vi "Stopped.vi"(6 "Teller":refnum<class "Teller.lvclass">, 8 "Error in":errorcluster, 9 "Error":errorcluster, 10 "Actor":refnum<class "Actor.lvclass">, 11 "Base Actor in":refnum<class "Base Actor.lvclass">) -> (0 "Error out":errorcluster, 3 "Base Actor out":refnum<class "Base Actor.lvclass">)   [LabVIEW 2025, in "jettl.lvlib" / "Base Actor.lvlib" / "Base Actor.lvclass"]
uses:
  Base Actor.lvclass
  C:/git/jettl/src/jettl/jettl/Actor/Actor.lvclass
  Actor/Actor.lvclass
  Teller/Teller.lvclass
  Base Actor.lvclass/Base Actor.ctl
  Stop jettl Msg/Call.vi
  Attributes/Attributes.lvclass
  C:/git/jettl/src/jettl/jettl/Base Actor/Base Actor/Base Actor.lvclass
  C:/git/jettl/src/jettl/jettl/Stop jettl Msg/Stop jettl Msg/Stop jettl Msg.lvclass
  C:/git/jettl/src/jettl/jettl/Stopped jettl Msg/Stopped/Stopped jettl Msg.lvclass
  Stop jettl Msg/Stop jettl Msg.lvlib
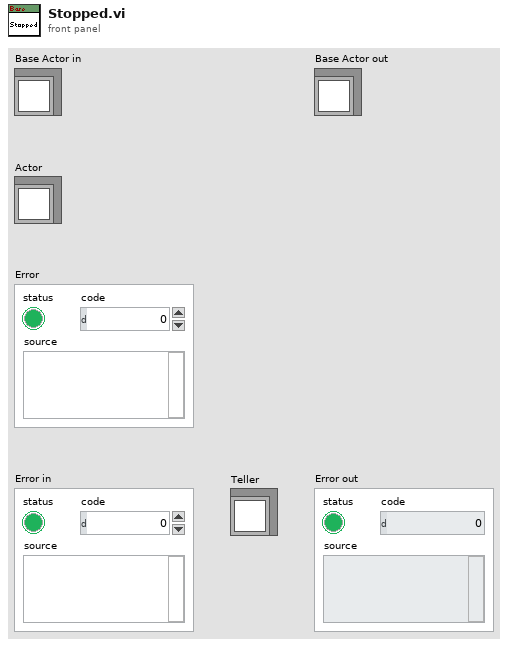
[diagram p1: front panel]
types:
  T1 = typedef "jettl.lvlib/Relation.ctl" = enum16{"Self", "Parent", "Child", "No Relation"}
  T2 = typedef "jettl.lvlib/All Child Attributes.ctl" = map{string, refnum<class "Attributes.lvclass">}
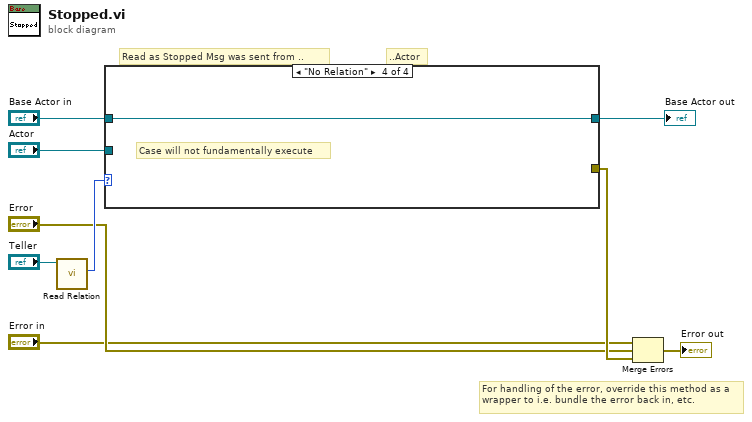
[diagram p0: block diagram]
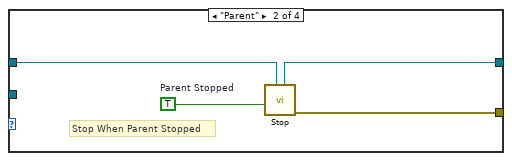
[diagram p3: hidden frame]
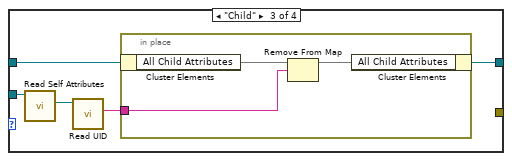
[diagram p4: hidden frame]
diagram:
  # "For handling of the error, override this method as a wrapper to i.e. bundle the error back in, etc."
  # "..Actor"
  # "Read as Stopped Msg was sent from .."
  n1 = call-dynamic "Read Relation.vi"("Teller in"="Teller") -> ("Relation"=w5:T1)  [unwired: 10 in]
  n2 = case shown="\"No Relation\"" w5 {
    tunnel: "Base Actor in" -> [w10 w12 w18 w23]
    tunnel: [w10 w14 w15 w23] -> w9
    tunnel: "Actor" -> [_ _ w19 _]
    tunnel: [_ w13 _ _] -> w3
    frame "Self" {
      # "Case will not fundamentally execute"
    }
    frame "Parent" {
      w11 = TRUE  # Parent Stopped
      # "Stop When Parent Stopped"
      n3 = call-poly "Stop.vi"("Actor in"=w12, "Parent Stopped"=w11) -> ("Error out"=w13:errorcluster, "Actor out"=w14:refnum<class "Base Actor.lvclass">)  [unwired: 8 in]
    }
    frame "Child" {
      n4 = call-dynamic "Read Self Attributes.vi"("Actor in"=w19) -> ("Self Attributes"=w17:refnum<class "Attributes.lvclass">)  [unwired: 10 in]
      n5 = call-dynamic "Read UID.vi"("Attributes in"=w17) -> ("UID"=w16:string)  [unwired: 10 in]
      n6 = in-place {
        in-place-border: w16 -> [w20]
        n7 = in-place-cluster #1(w18) -> ("All Child Attributes"=w22:T2)
        n8 = Remove From Map(10:w20, 11:w22) -> (3:w21:T2)  [unwired: 2 out]
        n9 = in-place-cluster #1("All Child Attributes"=w21) -> (w15:refnum<class "Base Actor.lvclass">)
      }
    }
    frame "No Relation" {
      # "Case will not fundamentally execute"
    }
  }
  "Base Actor out" <- w9
  n10 = Merge Errors("Error in", "Error", w3) -> (→"Error out":errorcluster)
